vi "Calculate Image Date.vi"(8 "error in (no error)":errorcluster, 10 "index":i32, 11 "Header in":refnum<class "Header.lvclass">) -> (0 "error out":errorcluster, 3 "Header out":refnum<class "Header.lvclass">)   [LabVIEW 2018, in "Header.lvclass"]
uses:
  Header.lvclass
  C:/Users/observer/Desktop/SPARC4_ACS/SPARC4_ACS/Simulated_Header/Simulated_Header.lvclass
  <vilib>/Utility/miscctls.llb/LVDateTimeRec.ctl
  Simulated_Header/Simulated_Header.lvclass
panel:
  in  "date time rec":T1
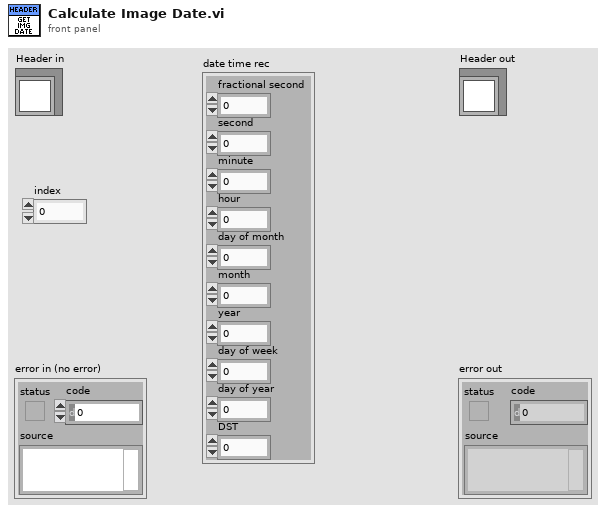
[diagram p1: front panel]
types:
  T1 = typedef "LVDateTimeRec.ctl" = cluster{"fractional second":dbl, "second":i32, "minute":i32, "hour":i32, "day of month":i32, "month":i32, "year":i32, "day of week":i32, "day of year":i32, "DST":i32}
  T2 = typedef "SYSTEMTIME structure typedef.ctl" = cluster{"Year":u16, "Month":u16, "DayOfWeek":u16, "Date":u16, "Hour":u16, "Minute":u16, "Second":u16, "Milliseconds":u16}
  T3 = cluster{"FILENAME":cluster{"Name":string, "Value":string, "Comment":string}, "OBSERVER":cluster{"Name":string, "Value":string, "Comment":string}, "PROGRID":cluster{"Name":string, "Value":string, "Comment":string}, "OBJECT":cluster{"Name":string, "Value":string, "Comment":string}, "NIGHTDIR":cluster{"Name":string, "Value":string, "Comment":string}, "CHANNEL":cluster{"Name":string, "Value":string, "Comment":string}, "INSTRUME":cluster{"Name":string, "Value":string, "Comment":string}, "NEXPSEQ":cluster{"Name":string, "Value":u16, "Comment":string}, "SEQINDEX":cluster{"Name":string, "Value":u16, "Comment":string}, "OBSTYPE":cluster{"Name":string, "Value":string, "Comment":string}, "READMOD":cluster{"Name":string, "Value":string, "Comment":string}, "READMODE":cluster{"Name":string, "Value":string, "Comment":string}, "ACQMODE":cluster{"Name":string, "Value":string, "Comment":string}, "PREAMP":cluster{"Name":string, "Value":string, "Comment":string}, "READOUT":cluster{"Name":string, "Value":string, "Comment":string}, "VSHIFT":cluster{"Name":string, "Value":string, "Comment":string}, "TRIGGER":cluster{"Name":string, "Value":string, "Comment":string}, "EMMODE":cluster{"Name":string, "Value":string, "Comment":string}, "EMGAIN":cluster{"Name":string, "Value":u16, "Comment":string}, "VBIN":cluster{"Name":string, "Value":u16, "Comment":string}, "HBIN":cluster{"Name":string, "Value":u16, "Comment":string}, "INITLIN":cluster{"Name":string, "Value":u16, "Comment":string}, "INITCOL":cluster{"Name":string, "Value":u16, "Comment":string}, "FINALLIN":cluster{"Name":string, "Value":u16, "Comment":string}, "FINALCOL":cluster{"Name":string, "Value":u16, "Comment":string}, "KSERLEN":cluster{"Name":string, "Value":u16, "Comment":string}, "SHUTTER":cluster{"Name":string, "Value":string, "Comment":string}, "OPENSHT":cluster{"Name":string, "Value":u16, "Comment":string}, "CLOSESHT":cluster{"Name":string, "Value":u16, "Comment":string}, "DATE":cluster{"Name":string, "Value":string, "Comment":string}, "GAIN":cluster{"Name":string, "Value":dbl, "Comment":string}, "GAINERR":cluster{"Name":string, "Value":dbl, "Comment":string}, "RDNOISE":cluster{"Name":string, "Value":dbl, "Comment":string}, "RNOISERR":cluster{"Name":string, "Value":dbl, "Comment":string}, "SKYFIBER":cluster{"Name":string, "Value":string, "Comment":string}, "CALFIBER":cluster{"Name":string, "Value":string, "Comment":string}, "UTDATE":cluster{"Name":string, "Value":string, "Comment":string}, "LOCTIME":cluster{"Name":string, "Value":string, "Comment":string}, "MJD":cluster{"Name":string, "Value":dbl, "Comment":string}, "OBSLON":cluster{"Name":string, "Value":string, "Comment":string}, "OBSLAT":cluster{"Name":string, "Value":string, "Comment":string}, "OBSALT":cluster{"Name":string, "Value":dbl, "Comment":string}, "EXPTIME":cluster{"Name":string, "Value":dbl, "Comment":string}, "TELRA":cluster{"Name":string, "Value":string, "Comment":string}, "TELDEC":cluster{"Name":string, "Value":string, "Comment":string}, "RA":cluster{"Name":string, "Value":string, "Comment":string}, "DEC":cluster{"Name":string, "Value":string, "Comment":string}, "RA_DEG":cluster{"Name":string, "Value":dbl, "Comment":string}, "DEC_DEG":cluster{"Name":string, "Value":dbl, "Comment":string}, "EPOCH":cluster{"Name":string, "Value":dbl, "Comment":string}, "HA":cluster{"Name":string, "Value":string, "Comment":string}, "HAD":cluster{"Name":string, "Value":dbl, "Comment":string}, "AIRMASS":cluster{"Name":string, "Value":dbl, "Comment":string}, "AMSTART":cluster{"Name":string, "Value":dbl, "Comment":string}, "AMEND":cluster{"Name":string, "Value":dbl, "Comment":string}, "XOFFSET":cluster{"Name":string, "Value":dbl, "Comment":string}, "YOFFSET":cluster{"Name":string, "Value":dbl, "Comment":string}, "PA":cluster{"Name":string, "Value":dbl, "Comment":string}, "CAMFOC":cluster{"Name":string, "Value":string, "Comment":string}, "TELFOC":cluster{"Name":string, "Value":dbl, "Comment":string}, "TCSUT":cluster{"Name":string, "Value":string, "Comment":string}, "TCSST":cluster{"Name":string, "Value":string, "Comment":string}, "MOONDIST":cluster{"Name":string, "Value":dbl, "Comment":string}, "MOONALT":cluster{"Name":string, "Value":dbl, "Comment":string}, "MOONPHAS":cluster{"Name":string, "Value":string, "Comment":string}, "ADC":cluster{"Name":string, "Value":string, "Comment":string}, "ADCSPEED":cluster{"Name":string, "Value":dbl, "Comment":string}, "CALMIRR":cluster{"Name":string, "Value":string, "Comment":string}, "GUIDING":cluster{"Name":string, "Value":string, "Comment":string}, "GUIDTEXP":cluster{"Name":string, "Value":dbl, "Comment":string}, "GUIDFREQ":cluster{"Name":string, "Value":dbl, "Comment":string}, "GUIDOBJX":cluster{"Name":string, "Value":dbl, "Comment":string}, "GUIDOBJY":cluster{"Name":string, "Value":dbl, "Comment":string}, "AVGYCORR":cluster{"Name":string, "Value":dbl, "Comment":string}, "AVGXCORR":cluster{"Name":string, "Value":dbl, "Comment":string}, "GFOCUS":cluster{"Name":string, "Value":dbl, "Comment":string}, "THARLAMP":cluster{"Name":string, "Value":string, "Comment":string}, "HALLAMP":cluster{"Name":string, "Value":string, "Comment":string}, "AGITATOR":cluster{"Name":string, "Value":string, "Comment":string}, "THARMIRR":cluster{"Name":string, "Value":string, "Comment":string}, "DSTATUS":cluster{"Name":string, "Value":string, "Comment":string}, "DPOS":cluster{"Name":string, "Value":dbl, "Comment":string}, "DTEMP":cluster{"Name":string, "Value":dbl, "Comment":string}, "DHUM":cluster{"Name":string, "Value":string, "Comment":string}, "DLAMP":cluster{"Name":string, "Value":string, "Comment":string}, "DFLAT":cluster{"Name":string, "Value":string, "Comment":string}, "TEMPEXT":cluster{"Name":string, "Value":string, "Comment":string}, "PRESSURE":cluster{"Name":string, "Value":string, "Comment":string}, "HUMIDITY":cluster{"Name":string, "Value":string, "Comment":string}, "WINDDIR":cluster{"Name":string, "Value":string, "Comment":string}, "WINSPEED":cluster{"Name":string, "Value":dbl, "Comment":string}, "SHTTTL":cluster{"Name":string, "Value":string, "Comment":string}, "COOLER":cluster{"Name":string, "Value":string, "Comment":string}, "TEMP":cluster{"Name":string, "Value":i16, "Comment":string}, "TEMPST":cluster{"Name":string, "Value":string, "Comment":string}, "SERN":cluster{"Name":string, "Value":u16, "Comment":string}, "COMMENT":cluster{"Name":string, "Value":string, "Comment":string}, "BITPIX":cluster{"Name":string, "Value":u16, "Comment":string}, "EXTEND":cluster{"Name":string, "Value":string, "Comment":string}, "FRAME_T":cluster{"Name":string, "Value":string, "Comment":string}, "VCLOCK":cluster{"Name":string, "Value":string, "Comment":string}, "ADCHNNL":cluster{"Name":string, "Value":u16, "Comment":string}, "JD":cluster{"Name":string, "Value":dbl, "Comment":string}, "SD":cluster{"Name":string, "Value":string, "Comment":string}, "FILTER":cluster{"Name":string, "Value":string, "Comment":string}, "ACSVRSN":cluster{"Name":string, "Value":string, "Comment":string}, "CTRLINTER":cluster{"Name":string, "Value":string, "Comment":string}, "TCSDATE":cluster{"TCSDATE":string, "Value":string, "Comment":string}}
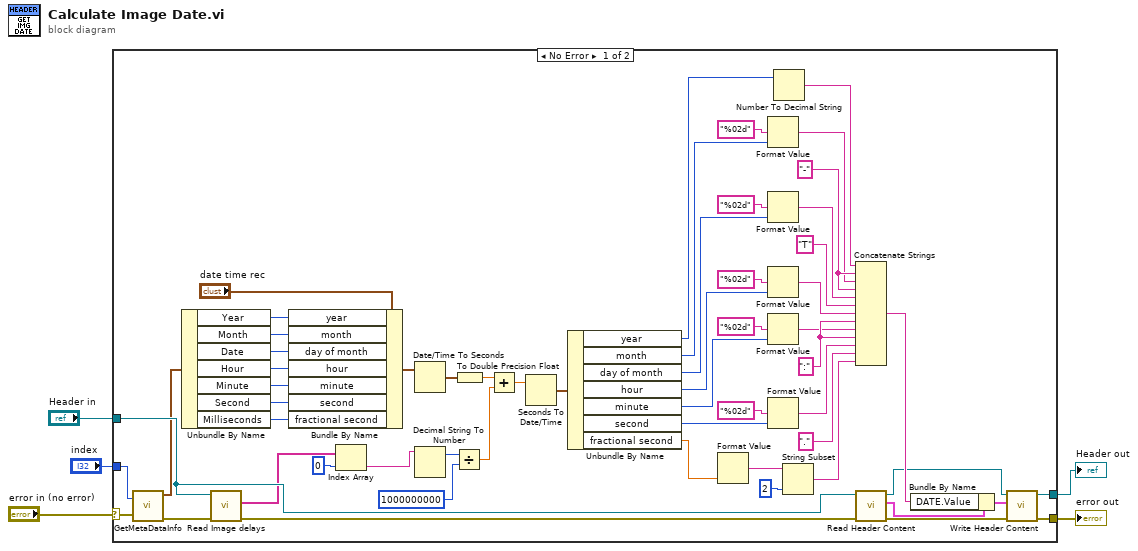
[diagram p0: block diagram]
diagram:
  n1 = case shown="No Error" "error in (no error)" {
    selector: "error in (no error)" -> [w37 w64]
    tunnel: [w41 w64] -> w3
    tunnel: [w40 w63] -> w2
    tunnel: "Header in" -> [w35 w63]
    tunnel: "index" -> [w36 _]
    frame No Error {
      w61 = ":"
      w62 = "-"
      n2 = call <userlib>:"GetMetaDataInfo.vi"("index"=w36, "error in (no error)"=w37) -> ("SYSTEMTIME"=w29:T2, "error out"=w34:errorcluster)  [unwired: 2 out]
      n3 = Unbundle By Name(w29) -> ("Year"=w28:u16, "Month"=w27:u16, "Date"=w26:u16, "Hour"=w25:u16, "Minute"=w24:u16, "Second"=w23:u16, "Milliseconds"=w22:u16)
      n4 = call "Read Image delays.vi"("error in (no error)"=w34, "Header in"=w35) -> ("error out"=w6:errorcluster, "Image delays"=w33:string[])  [unwired: 7 in, 1 out]
      n5 = Bundle By Name(cluster="date time rec", "year"=w28, "month"=w27, "day of month"=w26, "hour"=w25, "minute"=w24, "second"=w23, "fractional second"=w22) -> (w30:T1)
      n6 = Index Array(array=w33, index=0) -> (element=w20:string)
      n7 = Date/Time To Seconds(2:w30) -> (0:w21:timestamp)  [unwired: 1 in]
      n8 = Decimal String To Number(string=w20) -> (offset past number=w19:i32)  [unwired: 2 in, 1 out]
      n9 = Divide(x=w19, y=1000000000) -> (x/y=w16:dbl)
      n10 = To Double Precision Float(number=w21) -> (double precision float=w17:dbl)
      n11 = Add(x=w17, y=w16) -> (x+y=w15:dbl)
      n12 = Seconds To Date/Time(time stamp (now)=w15) -> (date time rec=w14:T1)  [unwired: 1 in]
      n13 = Unbundle By Name(w14) -> ("year"=w13:i32, "month"=w12:i32, "day of month"=w11:i32, "hour"=w10:i32, "minute"=w9:i32, "second"=w8:i32, "fractional second"=w7:dbl)
      n14 = Format Value(value (0)=w7) -> (output string=w54:string)  [unwired: 2 in]
      n15 = Format Value(format string="%02d", value (0)=w12) -> (output string=w52:string)  [unwired: 1 in]
      n16 = Format Value(format string="%02d", value (0)=w11) -> (output string=w51:string)  [unwired: 1 in]
      n17 = Format Value(format string="%02d", value (0)=w10) -> (output string=w49:string)  [unwired: 1 in]
      n18 = Format Value(format string="%02d", value (0)=w9) -> (output string=w48:string)  [unwired: 1 in]
      n19 = Format Value(format string="%02d", value (0)=w8) -> (output string=w47:string)  [unwired: 1 in]
      n20 = Number To Decimal String(number=w13) -> (decimal integer string=w53:string)  [unwired: 1 in]
      n21 = String Subset(string=w54, length (rest)=2 ("offset (0)")) -> (substring=w38:string)  [unwired: 1 in]
      n22 = Concatenate Strings(w53, w62, w52, w62, w51, "T", w49, w61, w48, w61, w47, ".", w38) -> (w46:string)
      n23 = call "Read Header Content.vi"("error in (no error)"=w6, "Simulated_Header in"=w35) -> ("error out"=w42:errorcluster, "Header Content"=w45:T3, "Simulated_Header out"=w44:refnum<class "Header.lvclass">)  [unwired: 7 in]
      n24 = Bundle By Name(cluster=w45, "DATE.Value"=w46) -> (w43:T3)
      n25 = call "Write Header Content.vi"("error in (no error)"=w42, "Header Content"=w43, "Simulated_Header in"=w44) -> ("error out"=w41:errorcluster, "Simulated_Header out"=w40:refnum<class "Header.lvclass">)  [unwired: 7 in]
    }
    frame Error {
    }
  }
  "error out" <- w3
  "Header out" <- w2
